vi "getFile.vi"(7 "isDir?":bool, 8 "error in (no error)":errorcluster, 9 "local path":path, 10 "remote path":string, 11 "ConnectionData":T1) -> (0 "error out":errorcluster, 3 "local path out":path)   [LabVIEW 2015]
uses:
  connectionData.ctl
panel:
  # "Gets a file from a remote location. Uses the pscp utility to perform the\ntransfer. This VI expects to find pscp.exe in the same dirctory that\nthis VI is located in.\nDOWNLOAD: http://www.chiark.greenend.org.uk/~sgtatham/putty/download.html"
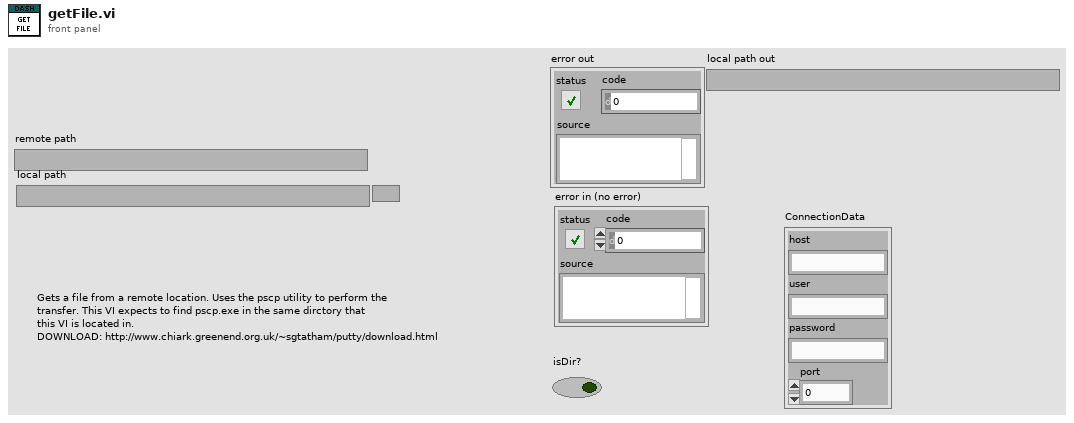
[diagram p1: front panel]
types:
  T1 = typedef "connectionData.ctl" = cluster{"host":string, "user":string, "password":string, "port":u16}
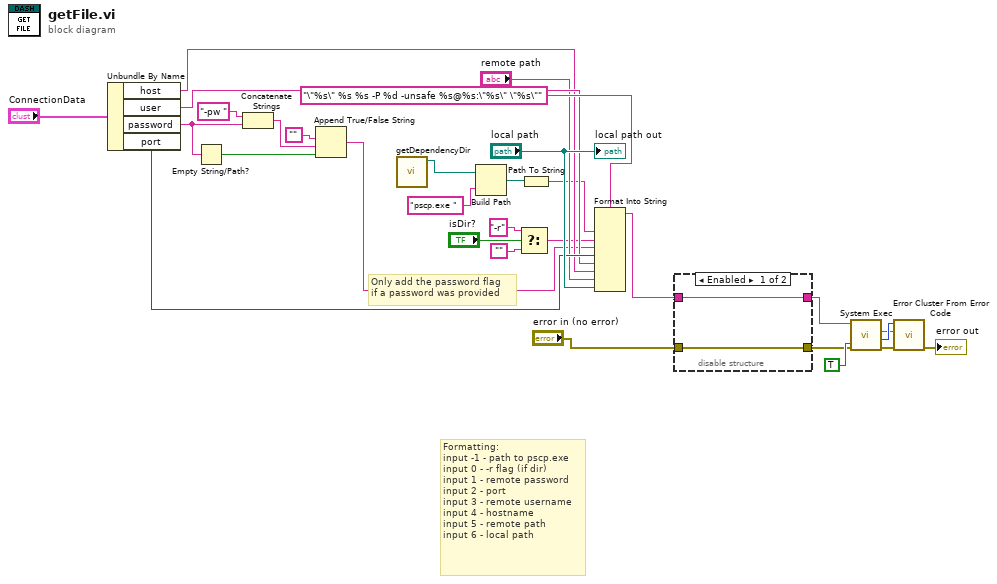
[diagram p0: block diagram]
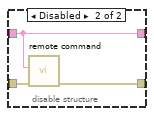
[diagram p2: hidden frame]
diagram:
  # "Only add the password flag\nif a password was provided"
  # "Formatting:\ninput -1 - path to pscp.exe\ninput 0 - -r flag (if dir)\ninput 1 - remote password\ninput 2 - port\ninput 3 - remote username\ninput 4 - hostname\ninput 5 - remote path\ninput 6 - local path"
  n1 = Unbundle By Name("ConnectionData") -> ("host"=w20:string, "user"=w21:string, "password"=w10:string, "port"=w22:u16)
  n2 = Empty String/Path?(string/path=w10) -> (empty?=w14:bool)
  n3 = Concatenate Strings("-pw " ("string"), w10) -> (w11:string)
  n4 = Append True/False String(1:w14, 2:w11, 3:"") -> (0:w9:string)  [unwired: 1 in]
  n5 = call "getDependencyDir.vi"() -> ("Dependency Directory"=w7:path)  [unwired: 11 in]
  n6 = Build Path(base path=w7, name or relative path="pscp.exe ") -> (appended path=w6:path)
  n7 = Select(t="-r", s="isDir?", f="") -> (s? t:f=w15:string)
  n8 = Path To String(path=w6) -> (string=w5:string)
  n9 = Format Into String(format string="\"%s\" %s %s -P %d -unsafe %s@%s:\"%s\" \"%s\"", w5, w15, w9, w22, w21, w20, "remote path", "local path") -> (resulting string=w4:string)  [unwired: 2 in, 1 out]
  n10 = disable-structure shown="Enabled" {
    disable-tunnel: w4 -> [w32 w33]
    disable-tunnel: "error in (no error)" -> [w31 w35]
    disable-tunnel: [w31 w34] -> w2
    disable-tunnel: [w32 w33] -> w1
    frame Enabled {
    }
    frame Disabled {
      n11 = call "remote command"("error in (no error)"=w35, "Message"=w33) -> ("error out"=w34:errorcluster)  [unwired: 8 in, 1 out]
    }
  }
  n12 = call <vilib>:"System Exec.vi"("run minimized? (F)"=TRUE, "error in (no error)"=w2, "command line"=w1) -> ("error out"=w27:errorcluster, "return code"=w29:i32, "standard error"=w28:string)  [unwired: 5 in, 1 out]
  n13 = call <vilib>:"Error Cluster From Error Code.vi"("error in (no error)"=w27, "error message (\"\")"=w28, "error code (0)"=w29) -> ("error out"=→"error out":errorcluster)  [unwired: 6 in]
  "local path out" <- "local path"
